vi "DI Search Channel.vi"(11 "DI Data":digitalwaveform[](array[waveform])) -> (3 "Array 2":bool[](array[boolean]))   [LabVIEW 2020]
uses:
  <vilib>/Waveform/DTblOps.llb/DTbl Digital to Boolean Array.vi
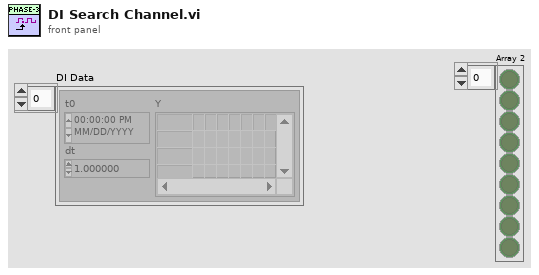
[diagram p1: front panel]
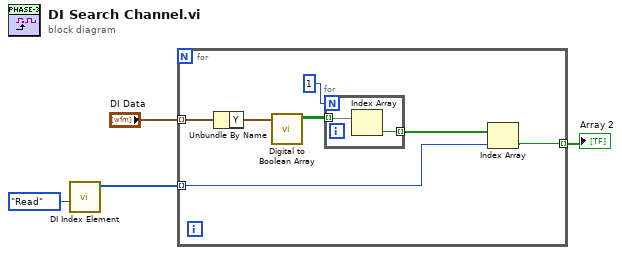
[diagram p0: block diagram]
diagram:
  n1 = call "DI Index Element.vi"("Write/Read"=enum16{"Write", "Read"}."Read") -> ("Index Element"=w1:i32[])  [unwired: 10 in]
  n2 = for {
    tunnel: "DI Data" -> [w8] mode=indexing
    tunnel: [w6] -> w3 mode=indexing
    tunnel: w1 -> [w5] mode=indexing
    n3 = Unbundle By Name(w8) -> ("Y"=w9:digitaldata)
    n4 = call-poly <vilib>:"Digital to Boolean Array.vi"("digital data"=w9) -> ("boolean array"=w10:bool[][])  [unwired: 9 in, 1 out]
    n5 = for {
      N: 1 -> [_]
      tunnel: w10 -> [w13] mode=indexing
      tunnel: [w12] -> w7 mode=indexing
      n6 = Index Array(array=w13) -> (element=w12:bool)  [unwired: 1 in]
    }
    n7 = Index Array(array=w7, index=w5) -> (element=w6:bool)
  }
  "Array 2" <- w3
